vi "Slope_WithError_#2.vi"(8 "Y2":dbl, 9 "X2":dbl, 10 "Y1":dbl, 11 "X1":dbl) -> (0 "?":string, 1 "Angle (Degrees)":dbl, 2 "Angle (Radians)":dbl, 3 "Linear Slope":dbl)   [LabVIEW 2020]
panel:
  out "error out":errorcluster
  in  "error in (no error)":errorcluster
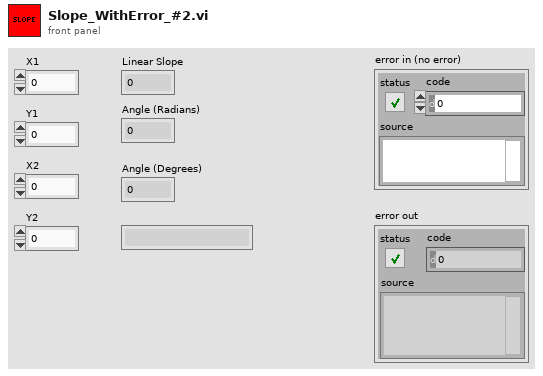
[diagram p1: front panel]
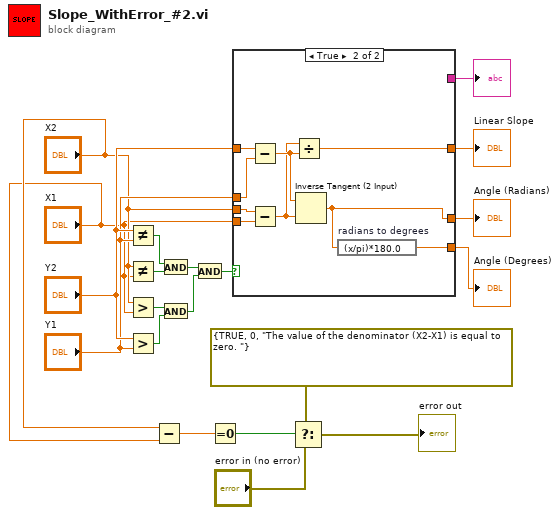
[diagram p0: block diagram]
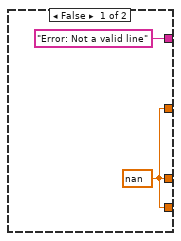
[diagram p2: hidden frame]
diagram:
  n1 = Not Equal?(x="Y2", y="Y1") -> (x != y?=w19:bool)
  n2 = Not Equal?(x="X2", y="X1") -> (x != y?=w18:bool)
  n3 = Greater?(x="X2", y="X1") -> (0:w14:bool)
  n4 = Greater?(x="Y2", y="Y1") -> (0:w10:bool)
  n5 = Subtract(x="X2", y="X1") -> (x-y=w5:dbl)
  n6 = And(x=w19, y=w18) -> (x .and. y?=w13:bool)
  n7 = And(x=w14, y=w10) -> (x .and. y?=w12:bool)
  n8 = And(x=w13, y=w12) -> (x .and. y?=w11:bool)
  n9 = Equal To 0?(x=w5) -> (x = 0?=w4:bool)
  n10 = case shown="True" w11 {
    tunnel: "Y1" -> [_ w31]
    tunnel: "Y2" -> [_ w30]
    tunnel: "X1" -> [_ w29]
    tunnel: "X2" -> [_ w28]
    tunnel: [w21 w27] -> w20
    tunnel: ["Error: Not a valid line" _] -> w17
    tunnel: [w21 w24] -> w16
    tunnel: [w21 w23] -> w15
    frame False {
      w21 = nan
    }
    frame True {
      n11 = Subtract(x=w30, y=w31) -> (x-y=w26:dbl)
      n12 = Subtract(x=w28, y=w29) -> (x-y=w25:dbl)
      n13 = Divide(x=w25, y=w26) -> (x/y=w27:dbl)
      n14 = Inverse Tangent (2 Input)(1:w25, 2:w26) -> (0:w24:dbl)
      n15 = expression code="(x/pi)*180.0" "radians to degrees"(w24) -> (w23:dbl)
    }
  }
  "Linear Slope" <- w20
  "?" <- w17
  "Angle (Radians)" <- w16
  "Angle (Degrees)" <- w15
  n16 = Select(t=errorcluster {TRUE, 0, "The value of the denominator (X2-X1) is equal to zero. "} ("error constant"), s=w4, f="error in (no error)") -> (s? t:f=→"error out":errorcluster)
